vi "Transient Capture - Arm Shot.vi"(8 "error in":errorcluster, 11 "Carrier Connection Out":T1) -> (0 "error out":errorcluster, 3 "DTACQ Connection Out":T1)   [LabVIEW 2017, in "Communications Library.lvlib"]
doc: "Sends the command to arm the transient shot, and waits until the device enters the armed state."
uses:
  Communications Library.lvlib
  Typedefs/DTACQ Connection Data--Cluster.ctl
  Typedefs/DTACQ Status--Enum.ctl
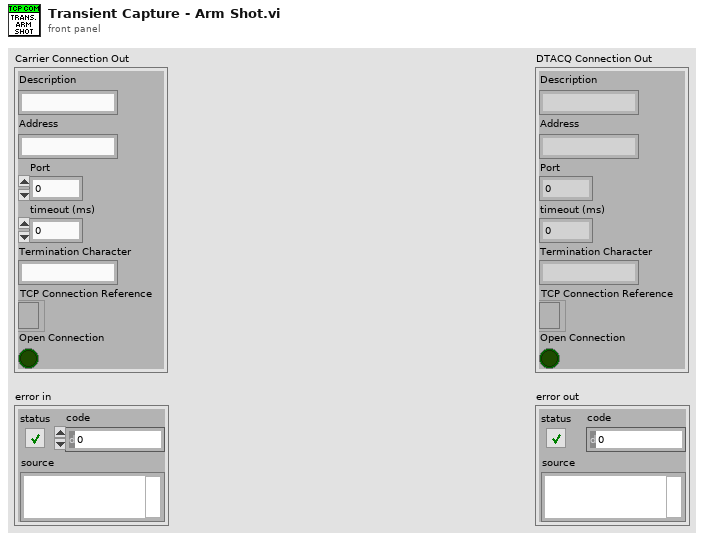
[diagram p1: front panel]
types:
  T1 = typedef "Communications Library.lvlib/DTACQ Connection Data--Cluster.ctl" = cluster{"Description":string, "Address":string, "Port":u16, "timeout (ms)":i32, "Termination Character":string, "TCP Connection Reference":refnum<k5>, "Open Connection":bool}
  T2 = typedef "Communications Library.lvlib/DTACQ Status--Enum.ctl" = enum16{"IDLE", "ARM", "RUN_PRE-TRIGGER", "RUN_POST-TRIGGER", "POST_PROCESS", "CLEANUP"}
  T3 = typedef "Communications Library.lvlib/DTACQ Module Carrier Status.ctl" = cluster{"DTACQ State":T2, "Pre-Trigger Samples":i32, "Post-Trigger Samples":i32, "Total Samples":i32, "Post Processing":bool}
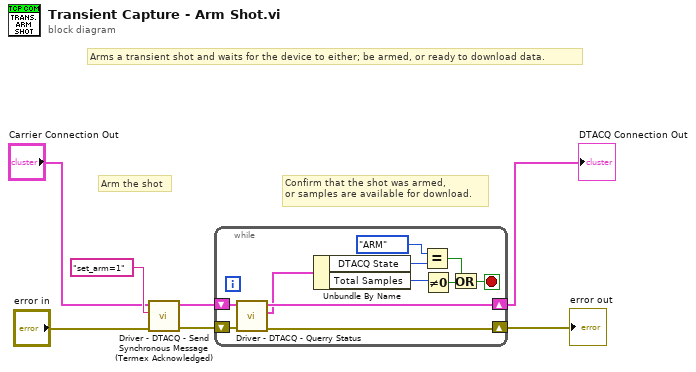
[diagram p0: block diagram]
diagram:
  # "Arms a transient shot and waits for the device to either; be armed, or ready to download data."
  # "Confirm that the shot was armed,\nor samples are available for download."
  # "Arm the shot"
  n1 = call "Driver - DTACQ - Send Synchronous Message (Termex Acknowledged).vi"("error in"="error in", "Message to Send"="set_arm=1", "DTACQ Connection Data In"="Carrier Connection Out") -> ("error out"=w1:errorcluster, "DTACQ Connection Data Out"=w2:T1)  [unwired: 5 in, 2 out]
  n2 = while {
    shift-right: [w15] -> w3
    shift-left: w2 -> [w17]
    shift-right: [w16] -> w4
    shift-left: w1 -> [w18]
    stop <- w8 stop-if-true
    n3 = call "Driver - DTACQ - Querry Status.vi"("error in"=w18, "DTACQ Connection Data In"=w17) -> ("error out"=w16:errorcluster, "Module Carrier Status"=w14:T3, "DTACQ Connection Data Out"=w15:T1)  [unwired: 6 in, 1 out]
    n4 = Unbundle By Name(w14) -> ("DTACQ State"=w13:T2, "Total Samples"=w11:i32)
    n5 = Equal?(x=DTACQ_Status--Enum."ARM", y=w13) -> (x = y?=w9:bool)
    n6 = Not Equal To 0?(x=w11) -> (x != 0?=w10:bool)
    n7 = Or(x=w9, y=w10) -> (x .or. y?=w8:bool)
  }
  "error out" <- w4
  "DTACQ Connection Out" <- w3
